vi "clearScanLog.vi"(8 "error in (no error)":errorcluster, 11 "Model in":refnum<class "Model.lvclass">) -> (0 "error out":errorcluster, 3 "Model out":refnum<class "Model.lvclass">)   [LabVIEW 2015, in "Model.lvclass"]
uses:
  Model.lvclass
  Model.lvclass/Model.ctl
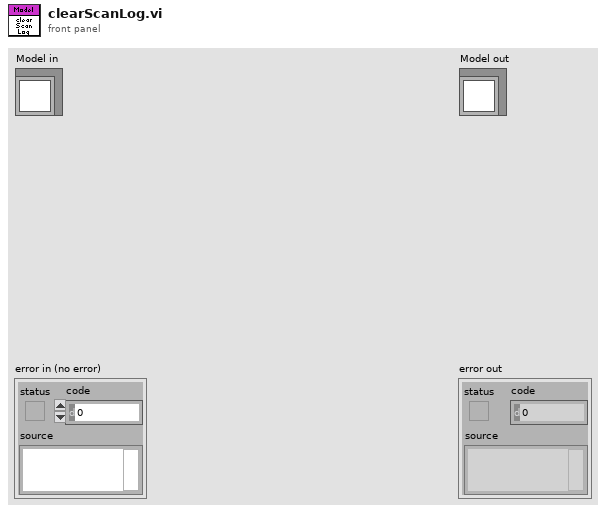
[diagram p1: front panel]
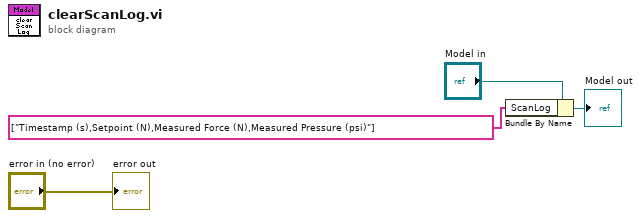
[diagram p0: block diagram]
diagram:
  n1 = Bundle By Name(cluster="Model in", "ScanLog"=string[] ["Timestamp (s),Setpoint (N),Measured Force (N),Measured Pressure (psi)"]) -> (→"Model out":refnum<class "Model.lvclass">)
  "error out" <- "error in (no error)"
